vi "mod_Create Continuous CPM.vi"(0 "Filter Length":i32, 1 "TX Filter":T2(ring), 5 "BT":dbl format="%.2f", 6 "error in (no error)":errorcluster, 7 "bits per symbol":i32, 8 "Symbol Rate, Hz":dbl format="%.2f", 9 "PN Sequence Order":i32, 10 "CPM system parameters":T1={"samples per symbol (16)"=16, "symbol map"=[]}) -> (2 "error out":errorcluster, 3 "samples per symbol":i32, 4 "output complex waveform":T3 {"Y" format="%.3f"; "dt" format="%^.2e"; "t0" format="%.4f"})   [LabVIEW 2020, in "niDMT.lvlib"]
uses:
  <vilib>/addons/Modulation/niDMT.lvlib
  <vilib>/addons/Modulation/Analog/controls/Complex Data Waveform.ctl
  <vilib>/addons/Modulation/Digital/Support/Controls/CPM System Parameters.ctl
  <vilib>/addons/Modulation/Analog/support/mod_Set Error Source.vi
  <vilib>/addons/Modulation/Digital/Support/Common/Validators/mod_Generate Filter Coefficients Validate.vi
  <vilib>/addons/Modulation/Digital/General/subVIs/mod_Generate Filter Coefficients.vi
  <vilib>/addons/Modulation/niAMT.lvlib
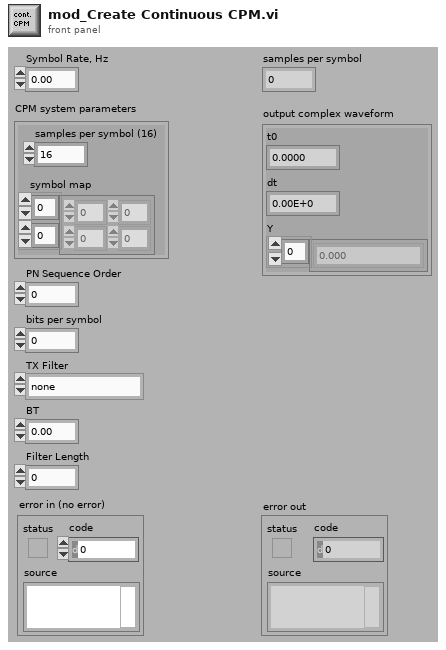
[diagram p1: front panel]
types:
  T1 = typedef "niDMT.lvlib/CPM System Parameters.ctl" = cluster{"samples per symbol (16)":i32, "symbol map":dbl[][]}
  T2 = enum16{"none", "Raised Cosine", "Root Raised Cos", "Gaussian"}
  T3 = typedef "niAMT.lvlib/Complex Data Waveform.ctl" = cluster{"t0":dbl, "dt":dbl, "Y":cdb[]}
  T4 = enum16{"FSK", "PSK", "QAM", "MSK", "PAM", "ASK", "CPM"}
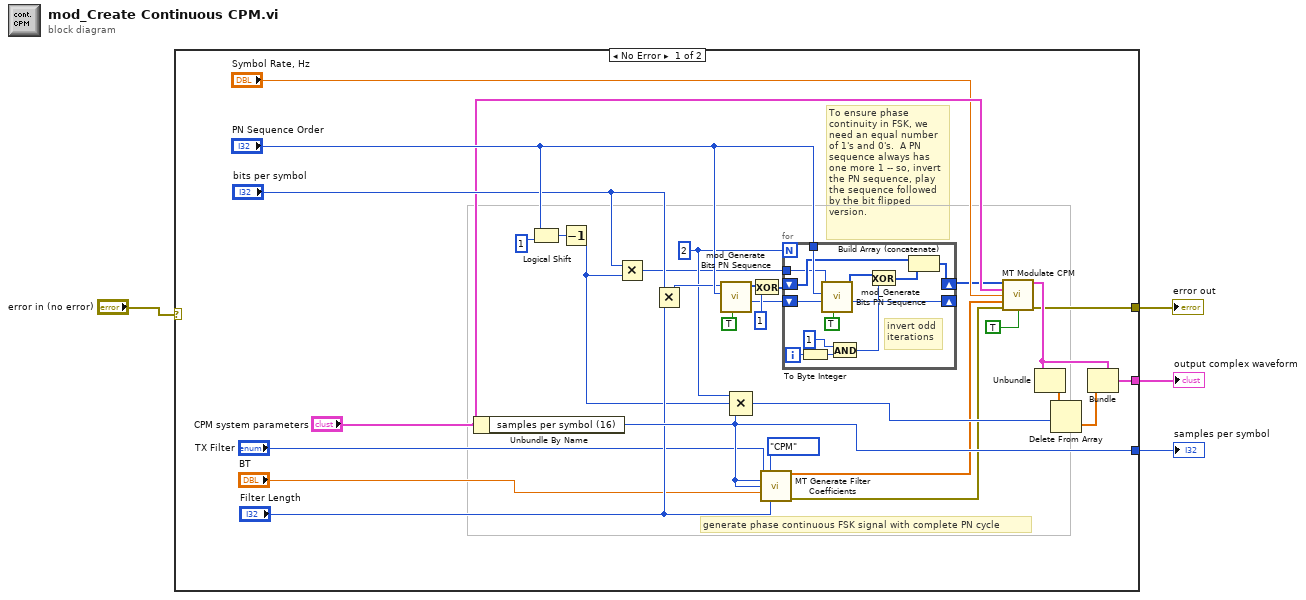
[diagram p0: block diagram]
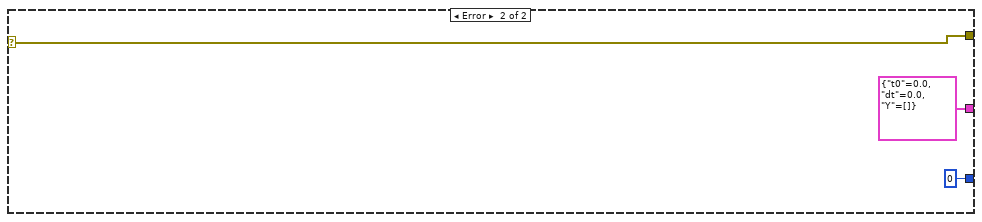
[diagram p2: hidden frame]
diagram:
  n1 = case shown="No Error" "error in (no error)" {
    selector: "error in (no error)" -> [_ w50]
    tunnel: [w7 w50] -> w4
    tunnel: [w34 cluster{"t0":dbl, "dt":dbl, "Y":cdb[]} {"t0"=0.0, "dt"=0.0, "Y"=[]} ("output complex waveform")] -> w3
    tunnel: [w32 0 ("samples per symbol (16)")] -> w2
    frame No Error {
      w15 = 2
      # "To ensure phase continuity in FSK, we need an equal number of 1's and 0's.  A PN sequence always has one more 1 -- so, invert the PN sequence, play the sequence followed by the bit flipped version."
      # "generate phase continuous FSK signal with complete PN cycle"
      n2 = Unbundle By Name("CPM system parameters") -> ("samples per symbol (16)"=w32:i32)
      n3 = Logical Shift(y="PN Sequence Order", x=1) -> (x << y=w19:i32)
      n4 = Decrement(x=w19) -> (x-1=w16:i32)
      n5 = Multiply(x="bits per symbol", y=w16) -> (x*y=w14:i32)
      n6 = Multiply(x="bits per symbol", y="Filter Length") -> (x*y=w25:i32)
      n7 = call <vilib>:"mod_Generate Bits PN Sequence.vi"("Reset? (T)"=TRUE ("Reset (T)"), "PN Sequence Order (9)"="PN Sequence Order", "Total Bits"=w25) -> ("seed out"=w26:u32, "Output Bit Stream"=w28:i8[])  [unwired: 1 in, 6 out]
      n8 = Compound Arithmetic op=MULTIPLY(w15, w16, w32) -> (w22:i32)
      n9 = Exclusive Or(1:i8 1 ("x"), 2:w28) -> (0:w30:i8[])
      n10 = call <vilib>:"MT Generate Filter Coefficients.vi"("pulse shaping filter (none)"="TX Filter", "modulation type"=T4."CPM", "pulse shaping samples per symbol (16)"=w32, "matched samples per symbol (16)"=w32, "filter parameter"="BT", "filter length (symbols)"="Filter Length") -> ("pulse shaping filter coefficients"=w11:dbl[], "error out"=w10:errorcluster)  [unwired: 1 in, 7 out]
      n11 = for {
        N: w15 -> [_]
        shift-right: [w46] -> _
        shift-left: w26 -> [w47]
        shift-right: [w43] -> w9
        shift-left: w30 -> [w42]
        tunnel: "PN Sequence Order" -> [w45]
        tunnel: w14 -> [w41]
        i -> [w39]
        # "invert odd\niterations"
        n12 = To Byte Integer(number=w39) -> (8bit integer=w35:i8)
        n13 = call <vilib>:"mod_Generate Bits PN Sequence.vi"("Reset? (T)"=TRUE ("Reset (T)"), "seed in (0xD6BF7DF2)"=w47, "PN Sequence Order (9)"=w45, "Total Bits"=w41) -> ("seed out"=w46:u32, "Output Bit Stream"=w44:i8[])  [unwired: 6 out]
        n14 = And(x=i8 1, y=w35) -> (x .and. y?=w36:i8)
        n15 = Exclusive Or(1:w36, 2:w44) -> (0:w37:i8[])
        n16 = Build Array (concatenate)(w42, w37) -> (w43:i8[])
      }
      n17 = call <vilib>:"MT Modulate CPM.vi"("input bit stream"=w9, "CPM system parameters"="CPM system parameters", "symbol rate (Hz)"="Symbol Rate, Hz", "pulse shaping filter coefficients"=w11, "error in (no error)"=w10, "reset? (T)"=TRUE ("Reset (T)")) -> ("output complex waveform"=w8:T3, "error out"=w7:errorcluster)  [unwired: 1 in, 7 out]
      n18 = Unbundle(w8) -> ("Y"=w21:cdb[])  [unwired: 2 out]
      n19 = Delete From Array(array=w21, length=w22) -> (deleted portion=w33:cdb[])  [unwired: 1 in, 1 out]
      n20 = Bundle(cluster=w8, "Y"=w33) -> (w34:T3)  [unwired: 2 out]
    }
    frame Error {
    }
  }
  "error out" <- w4
  "output complex waveform" <- w3
  "samples per symbol" <- w2
